vi "Write Token.vi"(8 "error in (no error)":errorcluster, 10 "Token":string, 11 "ByteGSWebAPI-V0 in":refnum<class "ByteGSWebAPI-V0.lvclass">) -> (0 "error out":errorcluster, 3 "ByteGSWebAPI-V0 out":refnum<class "ByteGSWebAPI-V0.lvclass">)   [LabVIEW 2019, in "ByteGSWebAPI-V0.lvclass"]
uses:
  ByteGSWebAPI-V0.lvclass
  ByteGSWebAPI-V0.lvclass/ByteGSWebAPI-V0.ctl
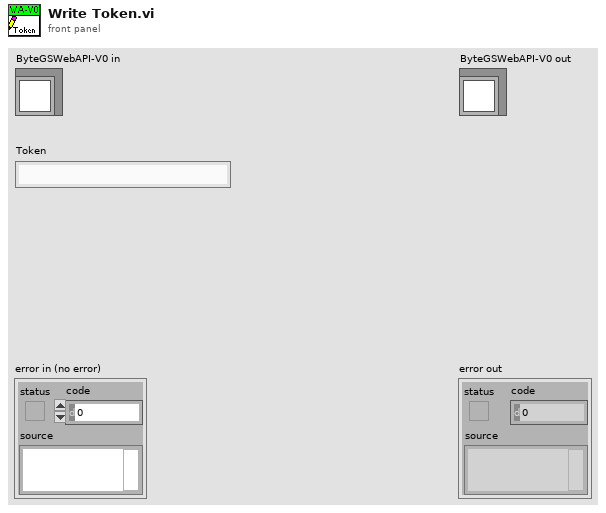
[diagram p1: front panel]
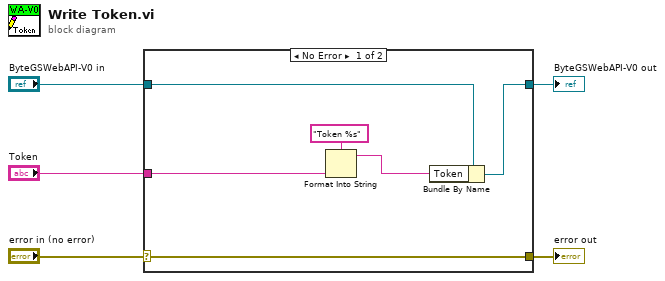
[diagram p0: block diagram]
diagram:
  n1 = case shown="No Error" "error in (no error)" {
    selector: "error in (no error)" -> [w11 w12]
    tunnel: [w11 w12] -> w4
    tunnel: [w9 w13] -> w2
    tunnel: "ByteGSWebAPI-V0 in" -> [w10 w13]
    tunnel: "Token" -> [w6 _]
    frame No Error {
      n2 = Format Into String(format string="Token %s", w6) -> (resulting string=w7:string)  [unwired: 2 in, 1 out]
      n3 = Bundle By Name(cluster=w10, "Token"=w7) -> (w9:refnum<class "ByteGSWebAPI-V0.lvclass">)
    }
    frame Error {
    }
  }
  "error out" <- w4
  "ByteGSWebAPI-V0 out" <- w2
